vi "OEE_SCREEN_2_build_worst_pace_array.vi"(11 "cycle_time_and_pace":string[][](array[string])) -> (3 "pace_from_worst":i32[][](array[numeric]))   [LabVIEW 2019]
uses:
  <userlib>/_OpenG.lib/array/array.llb/Filter 1D Array with Scalar (String)__ogtk.vi
  <userlib>/_OpenG.lib/array/array.llb/Delete Elements from 2D Array (String)__ogtk.vi
  <userlib>/_OpenG.lib/array/array.llb/Sort 2D Array (I32)__ogtk.vi
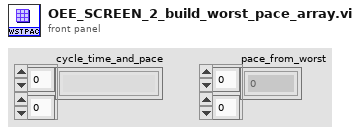
[diagram p1: front panel]
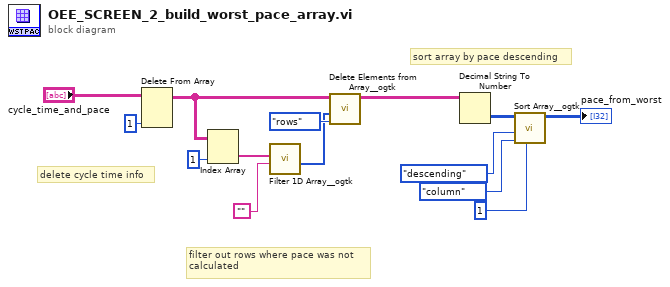
[diagram p0: block diagram]
diagram:
  # "sort array by pace descending"
  # "delete cycle time info"
  # "filter out rows where pace was not\ncalculated"
  n1 = Delete From Array(array="cycle_time_and_pace", index (col)=1 ("disabled index (col)")) -> (array with subset deleted=w13:string[][])  [unwired: 2 in, 1 out]
  n2 = Index Array(array=w13, index (col)=1 ("disabled index (col)")) -> (element=w7:string[])  [unwired: 1 in]
  n3 = call-poly <userlib>:"Filter 1D Array__ogtk.vi"("items to filter"="", "array"=w7) -> ("filtered item indices"=w9:i32[])  [unwired: 4 in, 1 out]
  n4 = call-poly <userlib>:"Delete Elements from Array__ogtk.vi"("delete (rows or columns)"=enum16{"rows", "columns"}."rows", "indices"=w9, "array"=w13) -> ("array w/ subset deleted"=w14:string[][])  [unwired: 7 in, 1 out]
  n5 = Decimal String To Number(string=w14) -> (number=w2:i32[][])  [unwired: 2 in, 1 out]
  n6 = call-poly <userlib>:"Sort Array__ogtk.vi"("Column/Row to Sort By"=u32 1, "Sort By in"=enum16{"row", "column"}."column", "Order"=enum16{"ascending", "descending"}."descending", "Array in"=w2) -> ("Sorted Array out"=→"pace_from_worst":i32[][])  [unwired: 4 in, 3 out]
